vi "Configure NRPM Measurement Frequency.vi"(6 "Frequency NRPM 3 (27.5GHz)":dbl=27500000000.0 format="%#.9p", 7 "Frequency NRPM 2 (27.5GHz)":dbl=27500000000.0 format="%#.9p", 8 "error in (no error)":errorcluster, 9 "Frequency NRPM 1 (27.5GHz)":dbl=27500000000.0 format="%#.9p", 10 "Instance (1)":i32=1, 11 "VISA resource name":refnum<visa-resource-name>) -> (0 "error out":errorcluster, 3 "VISA resource name out":refnum<visa-resource-name>)   [LabVIEW 2015, in "Rohde&Schwarz CMXP GPRF.lvlib"]
doc: "Specifies the input frequency at the power sensor connected to Sensor.\n\nAttribute:\nRSCMXPGPRF_ATTR_NRPM_MEASUREMENT_FREQUENCY\n\nRemote-control commands:\nCONFigure:GPRF:MEAS<i>:NRPM:SENSor1:FREQuency\nCONFigure:GPRF:MEAS<i>:NRPM:SENSor2:FREQuency\nCONFigure:GPRF:MEAS<i>:NRPM:SENSor3:FREQuency"
uses:
  <instrlib>/Rohde&Schwarz CMXP GPRF/Rohde&Schwarz CMXP GPRF.lvlib
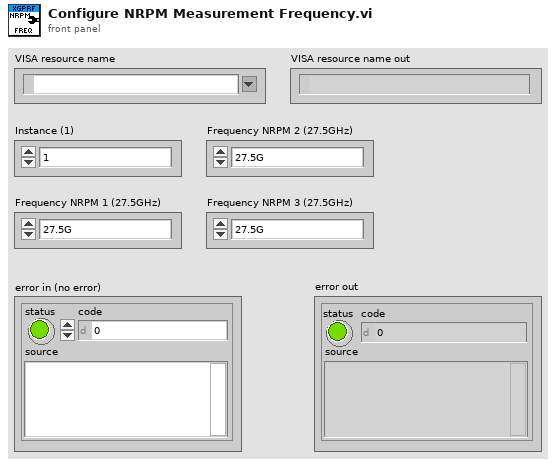
[diagram p1: front panel]
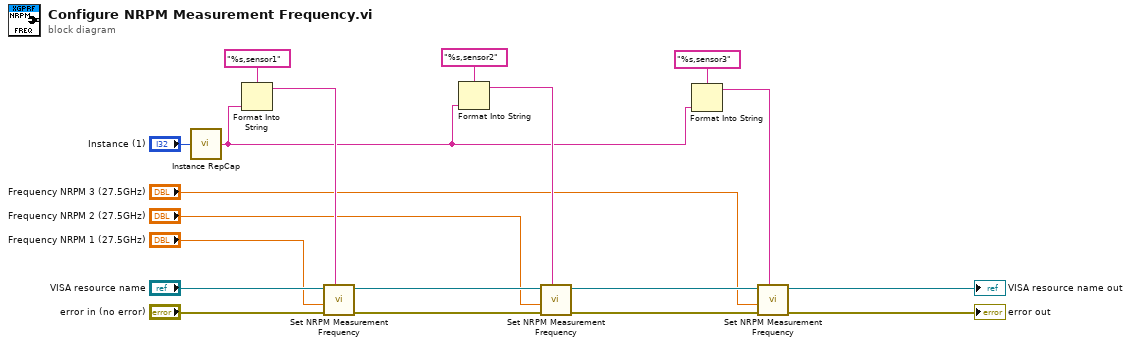
[diagram p0: block diagram]
diagram:
  n1 = call <instrlib>:"Instance RepCap.vi"("instance  in"="Instance (1)") -> ("instance out"=w5:string)
  n2 = Format Into String(format string="%s,sensor1", w5) -> (resulting string=w9:string)  [unwired: 2 in, 1 out]
  n3 = call "Set NRPM Measurement Frequency"("Repeated Capabilities"=w9, "error in (no error)"="error in (no error)", "NRPM Measurement Frequency (0.0)"="Frequency NRPM 1 (27.5GHz)", "instrument handle"="VISA resource name") -> ("error out"=w16:errorcluster, "instrument handle out"=w17:refnum<visa-resource-name>)  [unwired: 6 in]
  n4 = Format Into String(format string="%s,sensor2", w5) -> (resulting string=w7:string)  [unwired: 2 in, 1 out]
  n5 = call "Set NRPM Measurement Frequency"("Repeated Capabilities"=w7, "error in (no error)"=w16, "NRPM Measurement Frequency (0.0)"="Frequency NRPM 2 (27.5GHz)", "instrument handle"=w17) -> ("error out"=w12:errorcluster, "instrument handle out"=w13:refnum<visa-resource-name>)  [unwired: 6 in]
  n6 = Format Into String(format string="%s,sensor3", w5) -> (resulting string=w4:string)  [unwired: 2 in, 1 out]
  n7 = call "Set NRPM Measurement Frequency"("Repeated Capabilities"=w4, "error in (no error)"=w12, "NRPM Measurement Frequency (0.0)"="Frequency NRPM 3 (27.5GHz)", "instrument handle"=w13) -> ("error out"=→"error out":errorcluster, "instrument handle out"=→"VISA resource name out":refnum<visa-resource-name>)  [unwired: 6 in]
